vi "3.vi"() -> ()   [LabVIEW 2017]
panel:
  out "Thermometer":dbl(slide) scale=0.0..255.0
  out "Numeric":dbl
  in  "Array":bool[](array[boolean])
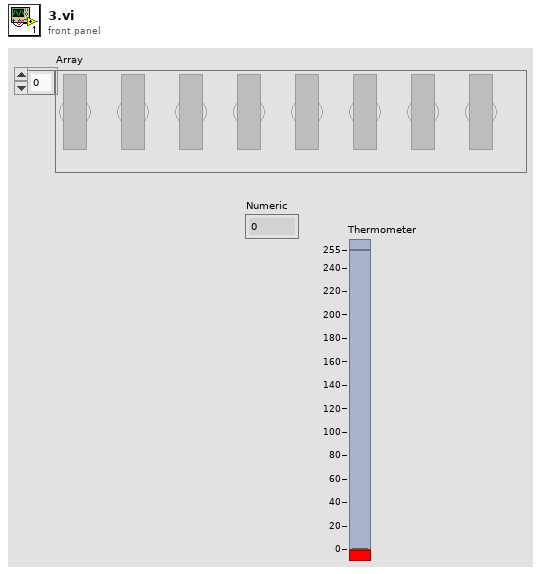
[diagram p1: front panel]
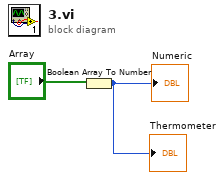
[diagram p0: block diagram]
diagram:
  n1 = Boolean Array To Number(Boolean array="Array") -> (number=→"Numeric" →"Thermometer":u32)
